vi "Increment Log Status.vi"(8 "error in":errorcluster, 10 "Trigger Received in":T1=enum."Start", 11 "Log Status Q in":refnum<queue>) -> (0 "error out":errorcluster, 2 "Trigger Received out":T1=enum."Start", 3 "Log Status Q out":refnum<queue>)   [LabVIEW 2015, in "Waveform Data Logger Engine.lvlib"]
uses:
  Waveform Data Logger Engine.lvlib
  Types/Log Status.ctl
  Types/Trigger Received.ctl
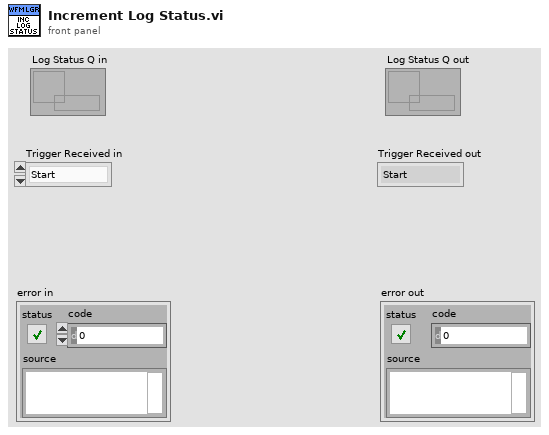
[diagram p1: front panel]
types:
  T1 = typedef "Waveform Data Logger Engine.lvlib/Trigger Received.ctl" = enum16{"None", "Start", "Stop", "Both", "Disable"}
  T2 = typedef "Waveform Data Logger Engine.lvlib/Log Status.ctl" = cluster{"Open Instances":i32, "Active Instances":i32, "Missed Samples":u64, "Error Code":i32}
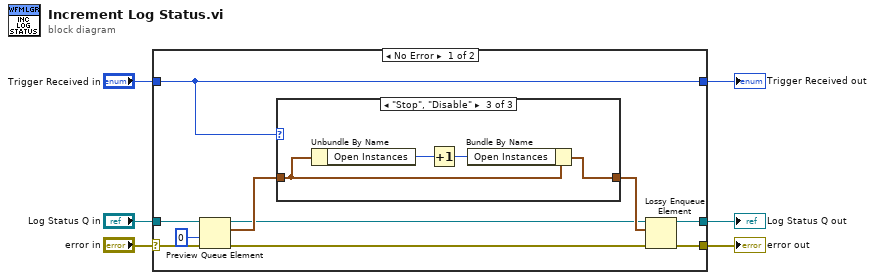
[diagram p0: block diagram]
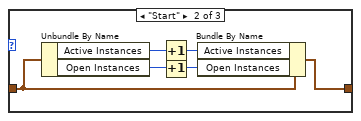
[diagram p3: hidden frame]
diagram:
  n1 = case shown="No Error" "error in" {
    selector: "error in" -> [w14 w28]
    tunnel: [w12 w30] -> w5
    tunnel: "Trigger Received in" -> [w12 w30]
    tunnel: "Log Status Q in" -> [w15 w29]
    tunnel: [w8 w29] -> w2
    tunnel: [w7 w28] -> w1
    frame No Error {
      n2 = Preview Queue Element(queue=w15, timeout in ms (-1)=0, error in (no error)=w14) -> (queue out=w10:refnum<queue>, element=w13:T2, error out=w9:errorcluster)  [unwired: 1 out]
      n3 = case shown="\"Stop\", \"Disable\"" w12 {
        tunnel: w13 -> [w17 w23 w27]
        tunnel: [w17 w18 w24] -> w11
        frame "None", Default {
        }
        frame "Start" {
          n4 = Unbundle By Name(w23) -> ("Active Instances"=w22:i32, "Open Instances"=w20:i32)
          n5 = Increment(x=w22) -> (x+1=w21:i32)
          n6 = Increment(x=w20) -> (x+1=w19:i32)
          n7 = Bundle By Name(cluster=w23, "Active Instances"=w21, "Open Instances"=w19) -> (w18:T2)
        }
        frame "Stop", "Disable" {
          n8 = Unbundle By Name(w27) -> ("Open Instances"=w26:i32)
          n9 = Increment(x=w26) -> (x+1=w25:i32)
          n10 = Bundle By Name(cluster=w27, "Open Instances"=w25) -> (w24:T2)
        }
      }
      n11 = Lossy Enqueue Element(queue=w10, element=w11, error in (no error)=w9) -> (queue out=w8:refnum<queue>, error out=w7:errorcluster)  [unwired: 2 out]
    }
    frame Error {
    }
  }
  "Log Status Q out" <- w2
  "error out" <- w1
  "Trigger Received out" <- w5
